vi "Core-DequeueCommands.vi"(8 "error in (no error)":errorcluster, 11 "Engine in":refnum<class "Engine.lvclass">) -> (0 "error out":errorcluster, 2 "Quit?":bool, 3 "Engine out":refnum<class "Engine.lvclass">)   [LabVIEW 2024, in "GLF.lvlib" / "Engine.lvclass"]
uses:
  Engine.lvclass
  Engine.lvclass/Engine.ctl
  Command-CreateDVR--cluster.ctl
  IAmGLF/IAmGLF.lvclass
  Command-DeleteDVR--cluster.ctl
  Command-RegisterWindow--cluster.ctl
  Window/Window.lvclass
  c534fc45-f9c2-42cc-8e01-6a6c0b1517e4.vi
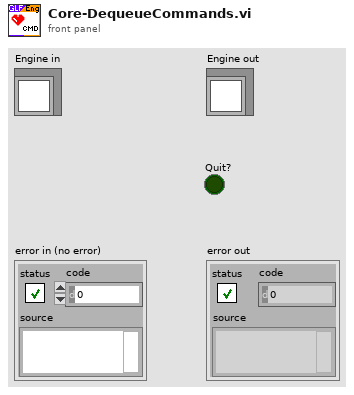
[diagram p1: front panel]
types:
  T1 = typedef "GLF.lvlib/Engine.lvclass/Command-CreateDVR--cluster.ctl" = cluster{"IAmGLF To Create DVR":refnum<class "IAmGLF.lvclass">, "IAmGLF Return Notifier":refnum<notifier>}
  T2 = typedef "GLF.lvlib/Engine.lvclass/Command-DeleteDVR--cluster.ctl" = cluster{"IAmGLF To Delete DVR":refnum<class "IAmGLF.lvclass">, "Error Return Notifier":refnum<notifier>}
  T3 = typedef "GLF.lvlib/Engine.lvclass/Command-RegisterWindow--cluster.ctl" = cluster{"Window":refnum<class "Window.lvclass">, "Error Return Notifier":refnum<notifier>}
  T4 = typedef "GLF.lvlib/Engine.lvclass/DVR--cluster.ctl" = cluster{"CMD Queue":T5, "Config":T6, "Ctxt":T8, "Metrics":T9, "GLF Instances":set{refnum<class "IAmGLF.lvclass">}, "Window Instances":map{i64, refnum<class "Window.lvclass">}}
  T5 = typedef "GLF.lvlib/Engine.lvclass/Command--queue.ctl" = refnum<queue>
  T6 = typedef "GLF.lvlib/Engine.lvclass/Config--cluster.ctl" = cluster{"Quit On Last Window Closed":bool, "VSync":T7, "FPS Target":dbl}
  T7 = typedef "GLF.lvlib/Engine.lvclass/VSync--enum.ctl" = enum16{"Disabled", "Enabled", "Adaptative"}
  T8 = typedef "GLF.lvlib/Engine.lvclass/Context--cluster.ctl" = cluster{"Ticks Begin":u64, "VSync Enabled":bool}
  T9 = typedef "GLF.lvlib/Engine.lvclass/Metrics--cluster.ctl" = cluster{"Uptime [ms]":u64, "Loop Time [ms]":u64}
  T10 = typedef "GLF.lvlib/Engine.lvclass/Command--cluster.ctl" = cluster{"Cmd":T11, "Data":variant}
  T11 = typedef "GLF.lvlib/Engine.lvclass/Command--enum.ctl" = enum16{"Quit", "Create DVR", "Delete DVR", "Register Window"}
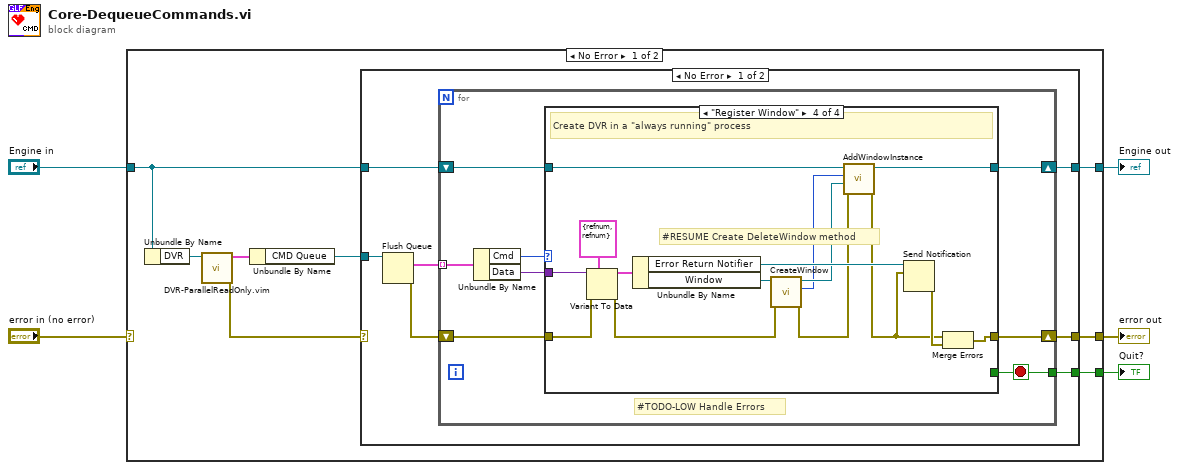
[diagram p0: block diagram]
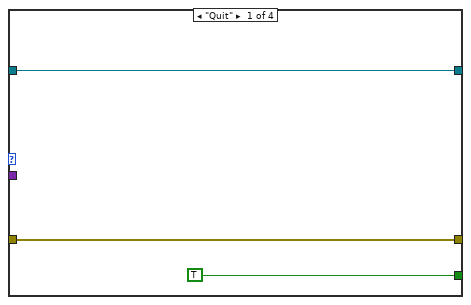
[diagram p2: hidden frame]
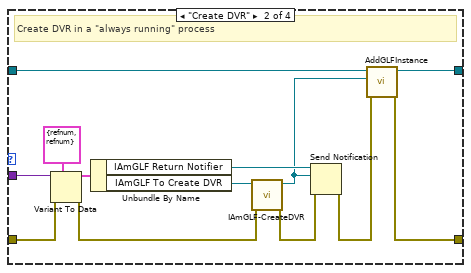
[diagram p3: hidden frame]
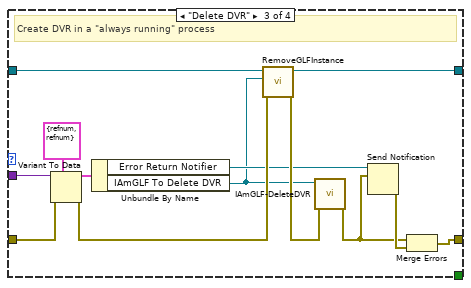
[diagram p4: hidden frame]
diagram:
  n1 = case shown="No Error" "error in (no error)" {
    selector: "error in (no error)" -> [_ w75]
    tunnel: [w11 w75] -> w4
    tunnel: [w10 _] -> w3
    tunnel: "Engine in" -> [w13 w76]
    tunnel: [w12 w76] -> w1
    frame No Error {
      n2 = Unbundle By Name(w13) -> ("DVR"=w9:refnum<data-value>)
      n3 = call "DVR-ParallelReadOnly.vim"("DVR"=w9) -> ("Error Out"=w7:errorcluster, "Data"=w8:T4)  [unwired: 9 in]
      n4 = Unbundle By Name(w8) -> ("CMD Queue"=w6:T5)
      n5 = case shown="No Error" w7 {
        selector: w7 -> [_ w73]
        tunnel: [w18 w73] -> w11
        tunnel: [w17 _] -> w10
        tunnel: w13 -> [w16 w74]
        tunnel: [w15 w74] -> w12
        tunnel: w6 -> [w14 _]
        frame No Error {
          n6 = Flush Queue(queue=w14) -> (remaining elements=w20:T10[], error out=w19:errorcluster)  [unwired: 1 in, 1 out]
          n7 = for {
            tunnel: w20 -> [w28] mode=indexing
            shift-right: [w26] -> w15
            shift-left: w16 -> [w27]
            shift-right: [w24] -> w18
            shift-left: w19 -> [w25]
            tunnel: [w22] -> w17
            stop <- w22 stop-if-true
            # "#TODO-LOW Handle Errors"
            n8 = Unbundle By Name(w28) -> ("Cmd"=w23:T11, "Data"=w21:variant)
            n9 = case shown="\"Register Window\"" w23 {
              tunnel: w27 -> [w31 w44 w55 w65]
              tunnel: [w31 w35 w50 w63] -> w26
              tunnel: w25 -> [w30 w43 w54 w72]
              tunnel: [w30 w33 w48 w68] -> w24
              tunnel: [TRUE _ _ _] -> w22
              tunnel: w21 -> [_ w42 w53 w71]
              frame "Quit" {
              }
              frame "Create DVR" {
                # "Create DVR in a \"always running\" process"
                n10 = Variant To Data(error in=w43, type=T1 {"IAmGLF To Create DVR"=refnum, "IAmGLF Return Notifier"=refnum} ("Data"), Variant=w42) -> (data=w40:T1, error out=w38:errorcluster)
                n11 = Unbundle By Name(w40) -> ("IAmGLF Return Notifier"=w37:refnum<notifier>, "IAmGLF To Create DVR"=w39:refnum<class "IAmGLF.lvclass">)
                n12 = call-dynamic "IAmGLF-CreateDVR.vi"("error in (no error)"=w38, "IAmGLF in"=w39) -> ("error out"=w36:errorcluster, "IAmGLF out"=w32:refnum<class "IAmGLF.lvclass">)  [unwired: 8 in]
                n13 = Send Notification(notification=w32, notifier=w37, error in (no error)=w36) -> (error out=w34:errorcluster)  [unwired: 1 out]
                n14 = call "AddGLFInstance.vi"("error in (no error)"=w34, "GLF Instance"=w32, "Engine in"=w44) -> ("error out"=w33:errorcluster, "Engine out"=w35:refnum<class "Engine.lvclass">)  [unwired: 7 in]
              }
              frame "Delete DVR" {
                # "Create DVR in a \"always running\" process"
                n15 = Variant To Data(error in=w54, type=T2 {"IAmGLF To Delete DVR"=refnum, "Error Return Notifier"=refnum} ("Data"), Variant=w53) -> (data=w52:T2, error out=w57:errorcluster)
                n16 = Unbundle By Name(w52) -> ("Error Return Notifier"=w51:refnum<notifier>, "IAmGLF To Delete DVR"=w46:refnum<class "IAmGLF.lvclass">)
                n17 = call "RemoveGLFInstance.vi"("error in (no error)"=w57, "GLF Instance"=w46, "Engine in"=w55) -> ("error out"=w56:errorcluster, "Engine out"=w50:refnum<class "Engine.lvclass">)  [unwired: 7 in]
                n18 = call-dynamic "IAmGLF-DeleteDVR.vi"("error in (no error)"=w56, "IAmGLF in"=w46) -> ("error out"=w45:errorcluster)  [unwired: 8 in, 1 out]
                n19 = Send Notification(notification=w45, notifier=w51) -> (error out=w47:errorcluster)  [unwired: 1 in, 1 out]
                n20 = Merge Errors(w45, w47) -> (w48:errorcluster)
              }
              frame "Register Window" {
                # "#RESUME Create DeleteWindow method"
                # "Create DVR in a \"always running\" process"
                n21 = Variant To Data(error in=w72, type=T3 {"Window"=refnum, "Error Return Notifier"=refnum} ("Data"), Variant=w71) -> (data=w70:T3, error out=w59:errorcluster)
                n22 = Unbundle By Name(w70) -> ("Error Return Notifier"=w69:refnum<notifier>, "Window"=w64:refnum<class "Window.lvclass">)
                n23 = call "CreateWindow.vi"("error in (no error)"=w59, "Window in"=w64) -> ("error out"=w58:errorcluster, "Window [SDL_Window *]"=w60:i64, "Window out"=w62:refnum<class "Window.lvclass">)  [unwired: 7 in]
                n24 = call "AddWindowInstance.vi"("error in (no error)"=w58, "Window Instance"=w62, "SDL_Window *"=w60, "Engine in"=w65) -> ("error out"=w61:errorcluster, "Engine out"=w63:refnum<class "Engine.lvclass">)  [unwired: 6 in]
                n25 = Send Notification(notification=w61, notifier=w69) -> (error out=w67:errorcluster)  [unwired: 1 in, 1 out]
                n26 = Merge Errors(w61, w67) -> (w68:errorcluster)
              }
            }
          }
        }
        frame Error {
        }
      }
    }
    frame Error {
    }
  }
  "error out" <- w4
  "Engine out" <- w1
  "Quit?" <- w3
